vi "Flock_Shared_Write Value to Local Process.vi"(8 "error in (no error)":errorcluster, 9 "Message Value":string, 10 "Message Name":string, 11 "Process List":T1) -> (0 "error out":errorcluster)   [LabVIEW 2014, in "Flock_Shared_Messaging.lvlib" / "Flock_Shared_LocalProcessMessaging.lvlib"]
uses:
  Flock_Shared_LocalProcessMessaging.lvlib
  FGV_Action.ctl
  Flock_Shared_Messaging.lvlib
  ProcessList.ctl
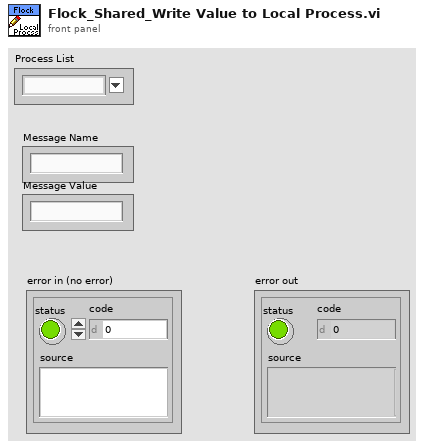
[diagram p1: front panel]
types:
  T1 = typedef "Flock_Shared_Messaging.lvlib/ProcessList.ctl" = string
  T2 = typedef "FGV_Action.ctl" = enum16{"Initalize Central", "Initialize Local", "Get", "Delete Local"}
  T3 = typedef "Flock_Shared_Messaging.lvlib/FGV_Queues.ctl" = cluster{"Local Queue in 2":T4, "Enum":T1}[]
  T4 = typedef "amc_Message Queue.ctl" = refnum<queue>
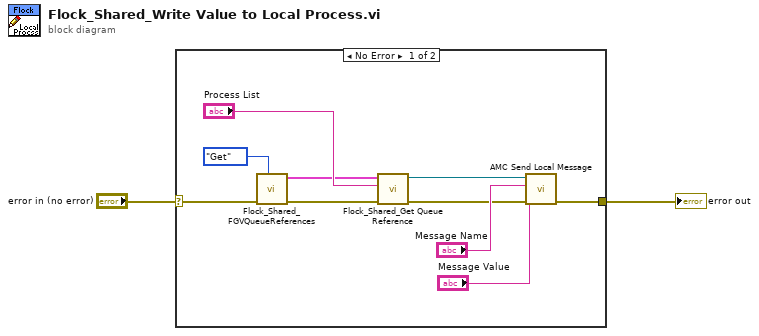
[diagram p0: block diagram]
diagram:
  n1 = case shown="No Error" "error in (no error)" {
    selector: "error in (no error)" -> [w9 w13]
    tunnel: [w12 w13] -> w2
    frame No Error {
      n2 = call "Flock_Shared_FGVQueueReferences.vi"("Action"=FGV_Action."Get", "error in (no error)"=w9) -> ("error out"=w6:errorcluster, "Array"=w3:T3)  [unwired: 7 in, 1 out]
      n3 = call "Flock_Shared_Get Queue Reference.vi"("Error In"=w6, "Enum"="Process List", "Array"=w3) -> ("Error Out"=w4:errorcluster, "Local Queue out"=w5:T4)  [unwired: 7 in]
      n4 = call <vilib>:"AMC Send Local Message.vi"("error in (no error)"=w4, "Message Value"="Message Value", "Message Name"="Message Name", "Message Queue in"=w5) -> ("error out"=w12:errorcluster)  [unwired: 6 in, 1 out]
    }
    frame Error {
    }
  }
  "error out" <- w2
